vi "Stop SubComponent.vi"(5 "Component ID":u8, 7 "FPGA Interface":refnum<class "FPGA Interface.lvclass">, 8 "error in (no error)":errorcluster, 11 "Remote Terminal in":refnum<class "Remote Terminal.lvclass">) -> (0 "error out":errorcluster, 3 "Remote Terminal out":refnum<class "Remote Terminal.lvclass">)   [LabVIEW 2020, in "BCI-1553 API.lvlib" / "Remote Terminal.lvclass"]
doc: "Disables this Remote Terminal, stops the operation of this Remote Terminal, and then re-enables this Remote Terminal."
uses:
  Remote Terminal.lvclass
  Dependencies/FPGA Interface/FPGA Interface.lvclass
  Remote Terminal.lvclass/Remote Terminal.ctl
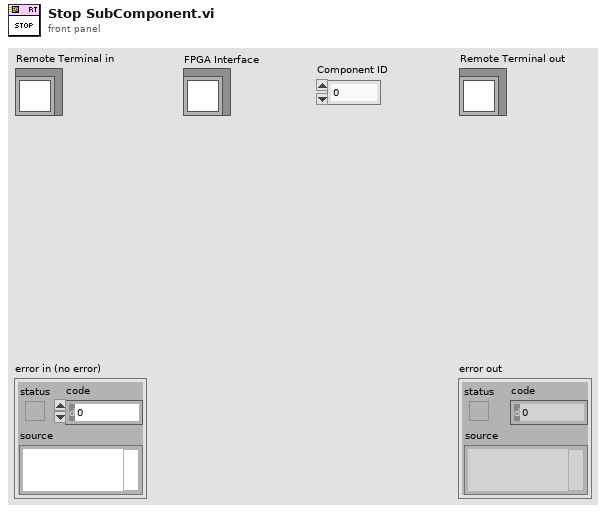
[diagram p1: front panel]
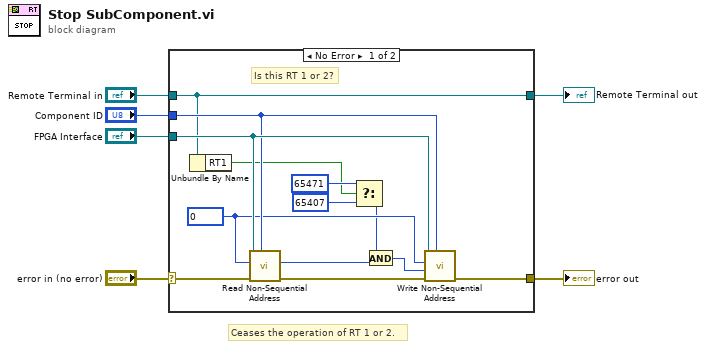
[diagram p0: block diagram]
diagram:
  # "Ceases the operation of RT 1 or 2."
  n1 = case shown="No Error" "error in (no error)" {
    selector: "error in (no error)" -> [w19 w21]
    tunnel: [w7 w21] -> w1
    tunnel: "Remote Terminal in" -> [w9 w20]
    tunnel: "FPGA Interface" -> [w16 _]
    tunnel: "Component ID" -> [w15 _]
    tunnel: [w9 w20] -> w2
    frame No Error {
      w14 = u16 0 ("Address")
      # "Is this RT 1 or 2?"
      n2 = Unbundle By Name(w9) -> ("RT1"=w8:bool)
      n3 = call-dynamic "Read Non-Sequential Address.vi"("Target IC (1-8)"=w15, "error in (no error)"=w19, "Address"=w14, "FPGA Interface in"=w16) -> ("error out"=w17:errorcluster, "Data"=w18:u16)  [unwired: 6 in]
      n4 = Select(t=u16 65471 ("Address"), s=w8, f=u16 65407 ("Address")) -> (s? t:f=w10:u16)
      n5 = And(x=w10, y=w18) -> (x .and. y?=w13:u16)
      n6 = call-dynamic "Write Non-Sequential Address.vi"("Target IC (1-8)"=w15, "error in (no error)"=w17, "Data"=w13, "Address"=w14, "FPGA Interface in"=w16) -> ("error out"=w7:errorcluster)  [unwired: 6 in]
    }
    frame Error {
    }
  }
  "error out" <- w1
  "Remote Terminal out" <- w2
